vi "IsThereEmergency.vi"(10 "Obstacle in front of us?":bool, 11 "Max Stay Force":dbl) -> (2 "Emergency Regime":T1, 3 "Is There An Emergency?":bool)   [LabVIEW 2013]
doc: "This VI should return 'TRUE' if the MB needs to go into emergency behavior. The two emergencies that we are leaving space for in the code right now are 1) going into No-Knockdown mode when high winds are sensed or 2) doing obstacle avoidance if (as of yet undetermined sensors) detect a dynamic obstacle.\n\nThis VI should also return the type of emergency, which will be used to set the reaction state.\n\nEric Schneider, Feb. 2014"
uses:
  Data/TypeDefs/Emergency Regimes.ctl
panel:
  # "PLACEHOLDER UNTIL THE SENSORS TO\nDETERMINE THESE THINGS ARE DONE"
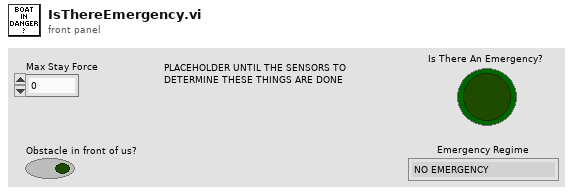
[diagram p1: front panel]
types:
  T1 = typedef "Emergency Regimes.ctl" = enum16{"NO EMERGENCY", "No Knockdown", "Obstacle Avoid"}
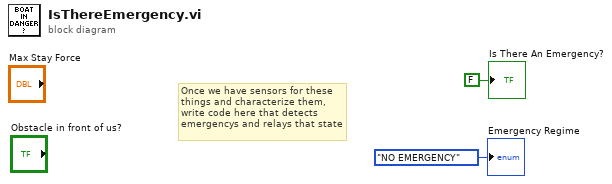
[diagram p0: block diagram]
diagram:
  # "Once we have sensors for these things and characterize them, write code here that detects emergencys and relays that state"
  "Is There An Emergency?" <- FALSE ("Is There An Emergency?")
  "Emergency Regime" <- Emergency_Regimes."NO EMERGENCY" ("Emergency Regimes")
